vi "Proton's Velocity.vi"(8 "Starting kinetic energy":dbl, 11 "Starting Velocity [optional]":dbl) -> (0 "Velocity (energy computed)":dbl, 3 "Velocity":dbl)   [LabVIEW 2020]
doc: "This SubVi computes velocity of proton using energy."
panel:
  # "This SubVi computes velocity in few ways"
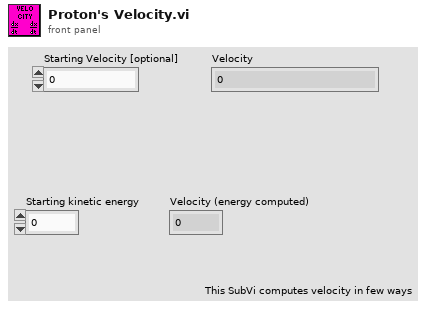
[diagram p1: front panel]
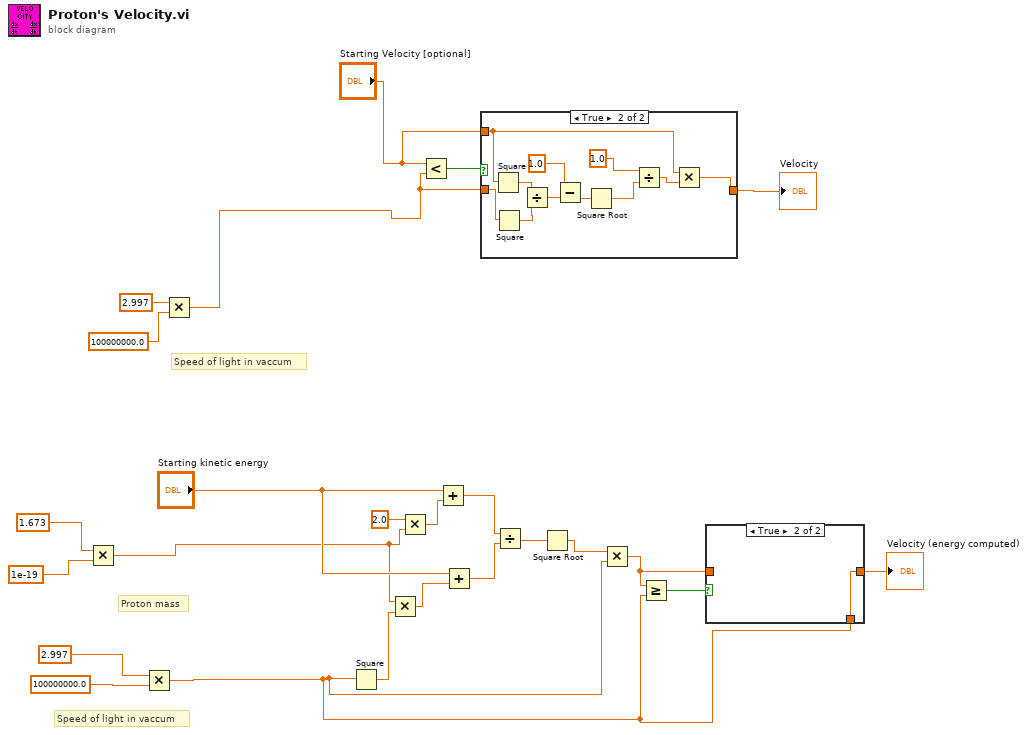
[diagram p0: block diagram]
diagram:
  # "Speed of light in vaccum"
  # "Proton mass"
  # "Speed of light in vaccum"
  n1 = Multiply(x=1.673, y=1e-19) -> (x*y=w1:dbl)
  n2 = Multiply(x=2.997, y=100000000.0) -> (x*y=w4:dbl)
  n3 = Multiply(x=2.997, y=100000000.0) -> (x*y=w7:dbl)
  n4 = Square(x=w4) -> (x^2=w18:dbl)
  n5 = Multiply(x=w1, y=w18) -> (x*y=w17:dbl)
  n6 = Multiply(x=2.0, y=w1) -> (x*y=w21:dbl)
  n7 = Less?(x="Starting Velocity [optional]", y=w7) -> (x < y?=w24:bool)
  n8 = Add(x="Starting kinetic energy", y=w21) -> (x+y=w16:dbl)
  n9 = Add(x="Starting kinetic energy", y=w17) -> (x+y=w15:dbl)
  n10 = case shown="True" w24 {
    tunnel: w7 -> [w25 w29]
    tunnel: [w25 w28] -> w23
    tunnel: "Starting Velocity [optional]" -> [_ w26]
    frame False {
    }
    frame True {
      n11 = Square(x=w26) -> (x^2=w32:dbl)
      n12 = Square(x=w29) -> (x^2=w30:dbl)
      n13 = Divide(x=w32, y=w30) -> (x/y=w31:dbl)
      n14 = Subtract(x=1.0, y=w31) -> (x-y=w34:dbl)
      n15 = Square Root(x=w34) -> (sqrt(x)=w35:dbl)
      n16 = Divide(x=1.0, y=w35) -> (x/y=w27:dbl)
      n17 = Multiply(x=w26, y=w27) -> (x*y=w28:dbl)
    }
  }
  "Velocity" <- w23
  n18 = Divide(x=w16, y=w15) -> (x/y=w14:dbl)
  n19 = Square Root(x=w14) -> (sqrt(x)=w13:dbl)
  n20 = Multiply(x=w13, y=w4) -> (x*y=w11:dbl)
  n21 = Greater Or Equal?(x=w11, y=w4) -> (x >= y?=w12:bool)
  n22 = case shown="True" w12 {
    tunnel: w11 -> [w37 _]
    tunnel: [w37 w38] -> w10
    tunnel: w4 -> [_ w38]
    frame False {
    }
    frame True {
    }
  }
  "Velocity (energy computed)" <- w10
